vi "CreateActionVI.vi"(6 "Agents class path":path, 8 "error in":errorcluster, 9 "VisitorFolder":path, 10 "VisitorClassPath":path, 11 "AgentsPublic":path) -> (0 "error out":errorcluster, 3 "actionVIPath":path)   [LabVIEW 2009, in "HGF_VisitorGenerator.lvlib"]
doc: "create visitors override action.vi, replace class controls, set to dynamic dispatch and replace agents public interface VI"
uses:
  HGF_VisitorGenerator.lvlib
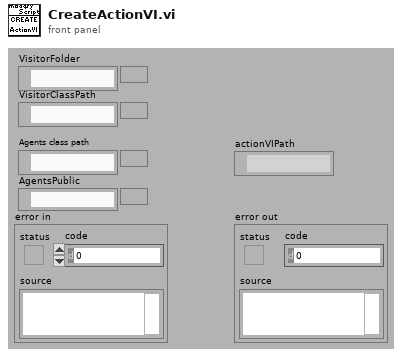
[diagram p1: front panel]
types:
  T1 = enum32{"invalid VI type", "Standard VI", "Control VI", "Global VI", "Polymorphic VI", "Configuration VI", "SubSystem", "Facade VI", "Method VI", "Statechart Diagram VI"}
  T2 = enum16{"Invalid Wire Rule", "Required", "Recommended", "Optional", "Dynamic Dispatch"}
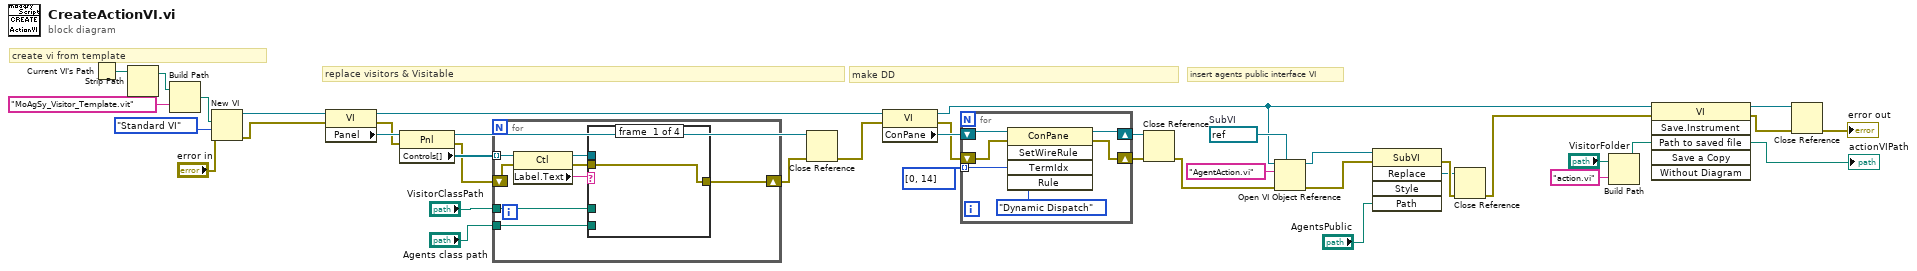
[diagram p0: block diagram]
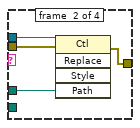
[diagram p2: hidden frame]
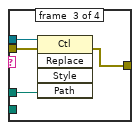
[diagram p3: hidden frame]
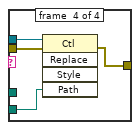
[diagram p4: hidden frame]
diagram:
  w15 = refnum<vi> refnum  # SubVI
  # "insert agents public interface VI"
  # "make DD"
  # "replace visitors & Visitable"
  # "create vi from template"
  n1 = Current VI's Path() -> (path=w4:path)
  n2 = Strip Path(path=w4) -> (stripped path=w1:path)  [unwired: 1 out]
  n3 = Build Path(base path=w1, name or relative path="MoAgSy_Visitor_Template.vit") -> (appended path=w2:path)
  n4 = New VI(8:"error in", 9:T1."Standard VI" ("vi type (standard vi)"), 10:w2) -> (0:w32:errorcluster, 3:w7:refnum<vi>)  [unwired: 4 in]
  n5 = property class="VI"(reference=w7, error in=w32) -> (reference out=w24:refnum<vi>, error out=w31:errorcluster, "Panel"=w33:refnum<vi>)
  n6 = property class="Pnl"(reference=w33, error in=w31) -> (reference out=w26:refnum<vi>, error out=w28:errorcluster, "Controls[]"=w30:refnum<vi>[])
  n7 = for {
    tunnel: w30 -> [w47] mode=indexing
    tunnel: "VisitorClassPath" -> [w45]
    shift-right: [w42] -> w27
    shift-left: w28 -> [w44]
    tunnel: "Agents class path" -> [w40]
    n8 = property class="Ctl"(reference=w47, error in=w44) -> (reference out=w46:refnum<vi>, error out=w43:errorcluster, "Label.Text"=w41:string)
    n9 = case shown="\"TC target\"" w41 {
      tunnel: w46 -> [_ w52 w56 w60]
      tunnel: w45 -> [_ w51 w53 _]
      tunnel: w43 -> [w48 w50 w54 w59]
      tunnel: [w48 w49 w55 w58] -> w42
      tunnel: w40 -> [_ _ _ w57]
      frame #0 {
      }
      frame #1 {
        n10 = invoke class="Ctl" method="Replace"(reference=w52, error in=w50, "Path"=w51) -> (error out=w49:errorcluster)  [unwired: 2 in, 4 out]
      }
      frame #2 {
        n11 = invoke class="Ctl" method="Replace"(reference=w56, error in=w54, "Path"=w53) -> (error out=w55:errorcluster)  [unwired: 2 in, 4 out]
      }
      frame #3 {
        n12 = invoke class="Ctl" method="Replace"(reference=w60, error in=w59, "Path"=w57) -> (error out=w58:errorcluster)  [unwired: 2 in, 4 out]
      }
    }
  }
  n13 = Close Reference(reference=w26, error in (no error)=w27) -> (error out=w22:errorcluster)
  n14 = property class="VI"(reference=w24, error in=w22) -> (reference out=w6:refnum<vi>, error out=w21:errorcluster, "ConPane"=w23:refnum<vi>)
  n15 = for {
    shift-right: [w63] -> w19
    shift-left: w21 -> [w64]
    shift-right: [w62] -> w20
    shift-left: w23 -> [w65]
    tunnel: u32[] [0, 14] -> [w61] mode=indexing
    n16 = invoke class="ConPane" method="SetWireRule"(reference=w65, error in=w64, "TermIdx"=w61, "Rule"=T2."Dynamic Dispatch") -> (reference out=w62:refnum<vi>, error out=w63:errorcluster)  [unwired: 1 in, 3 out]
  }
  n17 = Close Reference(reference=w20, error in (no error)=w19) -> (error out=w13:errorcluster)
  n18 = Open VI Object Reference(7:w15, 8:w13, 10:"AgentAction.vi" ("name/order"), 11:w6) -> (0:w11:errorcluster, 3:w12:refnum<vi>)
  n19 = invoke class="SubVI" method="Replace"(reference=w12, error in=w11, "Path"="AgentsPublic") -> (error out=w10:errorcluster, "Replace"=w9:refnum<vi>)  [unwired: 2 in, 3 out]
  n20 = Close Reference(reference=w9, error in (no error)=w10) -> (error out=w5:errorcluster)
  n21 = Build Path(base path="VisitorFolder", name or relative path="action.vi") -> (appended path=w34:path)
  "actionVIPath" <- w34
  n22 = invoke class="VI" method="Save.Instrument"(reference=w6, error in=w5, "Path to saved file"=w34) -> (reference out=w37:refnum<vi>, error out=w36:errorcluster)  [unwired: 3 in, 4 out]
  n23 = Close Reference(reference=w37, error in (no error)=w36) -> (error out=→"error out":errorcluster)
